vi "Start Acquisition.vi"(8 "error in (no error)":errorcluster, 11 "AutoExp in":refnum<class "AutoExp.lvclass">) -> (0 "error out":errorcluster, 3 "AutoExp out":refnum<class "AutoExp.lvclass">)   [LabVIEW 2018, in "AutoExp.lvclass"]
uses:
  AutoExp.lvclass
  AutoExp.lvclass/AutoExp.ctl
  State Machine/State Machine.lvclass
  TCS/TCS.lvclass
  Channel/Channel.lvclass
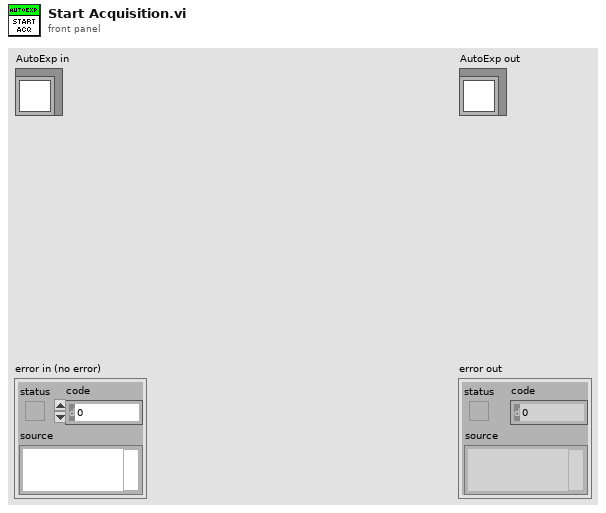
[diagram p1: front panel]
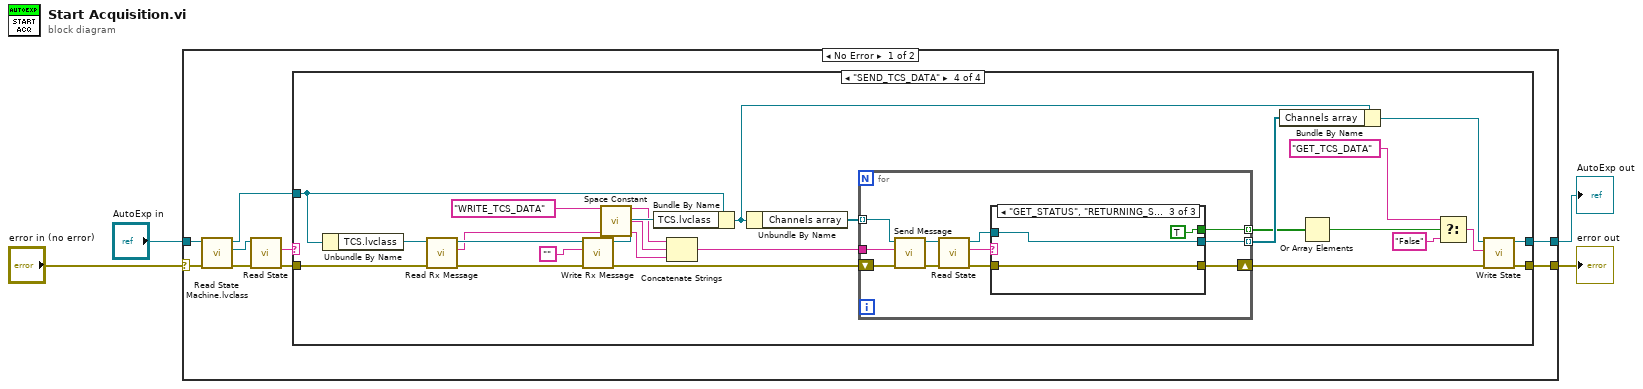
[diagram p0: block diagram]
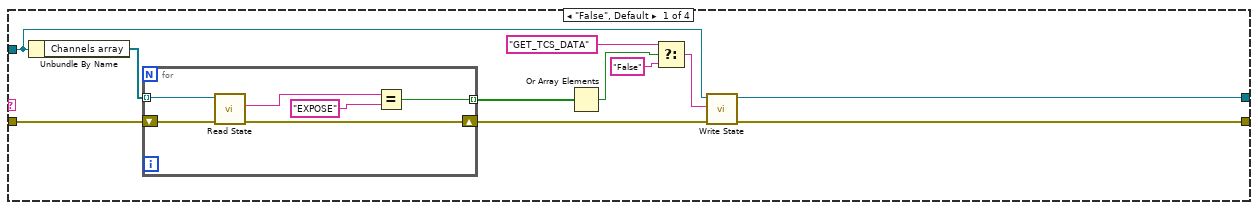
[diagram p2: hidden frame]
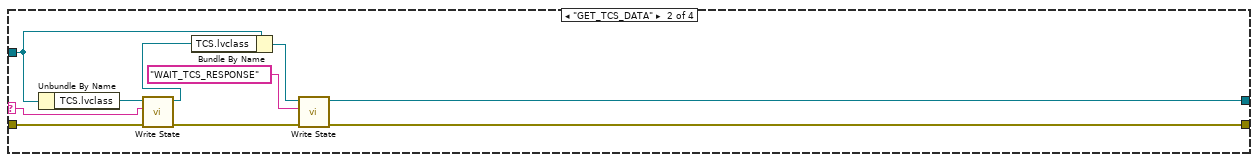
[diagram p3: hidden frame]
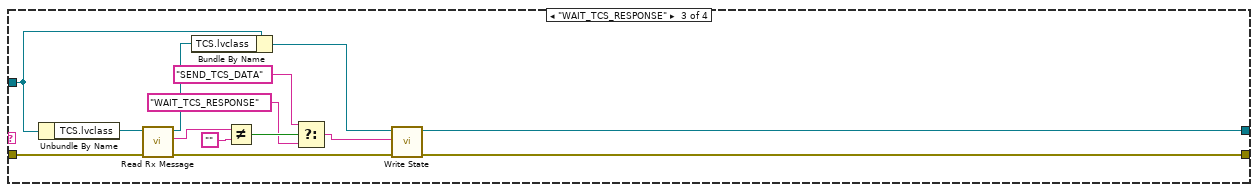
[diagram p4: hidden frame]
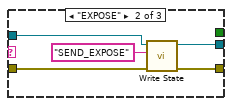
[diagram p6: hidden frame]
diagram:
  n1 = case shown="No Error" "error in (no error)" {
    selector: "error in (no error)" -> [w8 w101]
    tunnel: [w13 w101] -> w3
    tunnel: [w5 w100] -> w1
    tunnel: "AutoExp in" -> [w10 w100]
    frame No Error {
      n2 = call "Read State Machine.lvclass.vi"("error in (no error)"=w8, "AutoExp in"=w10) -> ("error out"=w9:errorcluster, "State Machine.lvclass"=w12:refnum<class "State Machine.lvclass">, "AutoExp out"=w11:refnum<class "AutoExp.lvclass">)  [unwired: 7 in]
      n3 = call-dynamic "Read State.vi"("error in (no error)"=w9, "State Machine in"=w12) -> ("error out"=w6:errorcluster, "State"=w7:string)  [unwired: 7 in, 1 out]
      n4 = case shown="\"SEND_TCS_DATA\"" w7 {
        selector: w7 -> [_ w40 _ _]
        tunnel: [w19 w33 w48 w65] -> w13
        tunnel: w11 -> [w21 w38 w53 w62]
        tunnel: w6 -> [w22 w36 w51 w63]
        tunnel: [w20 w34 w49 w60] -> w5
        frame "False", Default {
          n5 = Unbundle By Name(w21) -> ("Channels array"=w24:refnum<class "Channel.lvclass">[])
          n6 = for {
            tunnel: w24 -> [w30] mode=indexing
            shift-right: [w28] -> w18
            shift-left: w22 -> [w29]
            tunnel: [w25] -> w23 mode=indexing
            n7 = call "Read State.vi"("error in (no error)"=w29, "Channel in"=w30) -> ("error out"=w28:errorcluster, "State"=w27:string)  [unwired: 7 in, 1 out]
            n8 = Equal?(x=w27, y="EXPOSE") -> (x = y?=w25:bool)
          }
          n9 = Or Array Elements(Boolean array=w23) -> (logical OR=w14:bool)
          n10 = Select(t="GET_TCS_DATA" ("y"), s=w14, f="False" ("y")) -> (s? t:f=w17:string)
          n11 = call "Write State.vi"("error in (no error)"=w18, "State"=w17, "AutoExp in"=w21) -> ("error out"=w19:errorcluster, "AutoExp out"=w20:refnum<class "AutoExp.lvclass">)  [unwired: 7 in]
        }
        frame "GET_TCS_DATA" {
          n12 = Unbundle By Name(w38) -> ("TCS.lvclass"=w39:refnum<class "TCS.lvclass">)
          n13 = call "Write State.vi"("error in (no error)"=w36, "State"=w40, "TCS in"=w39) -> ("error out"=w32:errorcluster, "TCS out"=w37:refnum<class "TCS.lvclass">)  [unwired: 7 in]
          n14 = Bundle By Name(cluster=w38, "TCS.lvclass"=w37) -> (w35:refnum<class "AutoExp.lvclass">)
          n15 = call "Write State.vi"("error in (no error)"=w32, "State"="WAIT_TCS_RESPONSE", "AutoExp in"=w35) -> ("error out"=w33:errorcluster, "AutoExp out"=w34:refnum<class "AutoExp.lvclass">)  [unwired: 7 in]
        }
        frame "WAIT_TCS_RESPONSE" {
          n16 = Unbundle By Name(w53) -> ("TCS.lvclass"=w54:refnum<class "TCS.lvclass">)
          n17 = call "Read Rx Message.vi"("error in (no error)"=w51, "TCS in"=w54) -> ("error out"=w47:errorcluster, "Rx message"=w46:string, "TCS out"=w52:refnum<class "TCS.lvclass">)  [unwired: 7 in]
          n18 = Bundle By Name(cluster=w53, "TCS.lvclass"=w52) -> (w50:refnum<class "AutoExp.lvclass">)
          n19 = Not Equal?(x=w46, y="") -> (x != y?=w45:bool)
          n20 = Select(t="SEND_TCS_DATA", s=w45, f="WAIT_TCS_RESPONSE") -> (s? t:f=w42:string)
          n21 = call "Write State.vi"("error in (no error)"=w47, "State"=w42, "AutoExp in"=w50) -> ("error out"=w48:errorcluster, "AutoExp out"=w49:refnum<class "AutoExp.lvclass">)  [unwired: 7 in]
        }
        frame "SEND_TCS_DATA" {
          n22 = Unbundle By Name(w62) -> ("TCS.lvclass"=w64:refnum<class "TCS.lvclass">)
          n23 = call "Read Rx Message.vi"("error in (no error)"=w63, "TCS in"=w64) -> ("error out"=w71:errorcluster, "Rx message"=w69:string, "TCS out"=w70:refnum<class "TCS.lvclass">)  [unwired: 7 in]
          n24 = call "Write Rx Message.vi"("error in (no error)"=w71, "Rx message"="", "TCS in"=w70) -> ("error out"=w75:errorcluster, "TCS out"=w72:refnum<class "TCS.lvclass">)  [unwired: 7 in]
          n25 = call <vilib>:"Space Constant.vi"() -> ("String"=w68:string)
          n26 = Bundle By Name(cluster=w62, "TCS.lvclass"=w72) -> (w76:refnum<class "AutoExp.lvclass">)
          n27 = Concatenate Strings("WRITE_TCS_DATA", w68, w69) -> (w74:string)
          n28 = Unbundle By Name(w76) -> ("Channels array"=w73:refnum<class "Channel.lvclass">[])
          n29 = for {
            tunnel: w73 -> [w85] mode=indexing
            tunnel: [w87] -> w77 mode=indexing
            tunnel: w74 -> [w88]
            shift-right: [w86] -> w78
            shift-left: w75 -> [w89]
            tunnel: [w79] -> w59 mode=indexing
            n30 = call "Send Message.vi"("error in (no error)"=w89, "message"=w88, "Channel in"=w85) -> ("error out"=w83:errorcluster, "Channel out"=w84:refnum<class "Channel.lvclass">)  [unwired: 7 in]
            n31 = call "Read State.vi"("error in (no error)"=w83, "Channel in"=w84) -> ("error out"=w81:errorcluster, "State"=w80:string, "Channel out"=w82:refnum<class "Channel.lvclass">)  [unwired: 7 in]
            n32 = case shown="\"GET_STATUS\", \"RETURNING_STATUS\", \"WAIT_STATUS\"" w80 {
              tunnel: [w91 w96 w99] -> w87
              tunnel: [w90 w95 w98] -> w86
              tunnel: w82 -> [w91 w93 w99]
              tunnel: w81 -> [w90 w92 w98]
              tunnel: [_ _ TRUE] -> w79
              frame "False", Default {
              }
              frame "EXPOSE" {
                n33 = call "Write State.vi"("error in (no error)"=w92, "State"="SEND_EXPOSE", "Channel in"=w93) -> ("error out"=w95:errorcluster, "Channel out"=w96:refnum<class "Channel.lvclass">)  [unwired: 7 in]
              }
              frame "GET_STATUS", "RETURNING_STATUS", "WAIT_STATUS" {
              }
            }
          }
          n34 = Bundle By Name(cluster=w76, "Channels array"=w77) -> (w61:refnum<class "AutoExp.lvclass">)
          n35 = Or Array Elements(Boolean array=w59) -> (logical OR=w57:bool)
          n36 = Select(t="GET_TCS_DATA", s=w57, f="False") -> (s? t:f=w56:string)
          n37 = call "Write State.vi"("error in (no error)"=w78, "State"=w56, "AutoExp in"=w61) -> ("error out"=w65:errorcluster, "AutoExp out"=w60:refnum<class "AutoExp.lvclass">)  [unwired: 7 in]
        }
      }
    }
    frame Error {
    }
  }
  "error out" <- w3
  "AutoExp out" <- w1
